vi "Set_Offset_dir.vi"(2 "DEC":dbl, 3 "RA":dbl) -> (0 "DEC_dir":string, 1 "RA_dir":string)   [LabVIEW 2011]
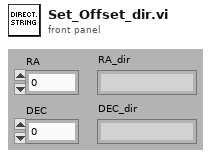
[diagram p1: front panel]
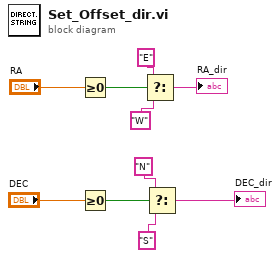
[diagram p0: block diagram]
diagram:
  n1 = Greater Or Equal To 0?(x="RA") -> (x >= 0?=w7:bool)
  n2 = Greater Or Equal To 0?(x="DEC") -> (x >= 0?=w8:bool)
  n3 = Select(t="E", s=w7, f="W") -> (s? t:f=→"RA_dir":string)
  n4 = Select(t="N", s=w8, f="S") -> (s? t:f=→"DEC_dir":string)
